vi "PopupList.vi"(8 "error in (no error)":errorcluster, 11 "BreadcrumbNavigation in":refnum<class "BreadcrumbNavigator.lvclass">) -> (0 "error out":errorcluster, 2 "SelectedItem":string, 3 "BreadcrumbNavigation out":refnum<class "BreadcrumbNavigator.lvclass">)   [LabVIEW 2015, in "BreadcrumbNavigator.lvclass"]
uses:
  BreadcrumbNavigator.lvclass
  <vilib>/Utility/miscctls.llb/LVPointTypeDef.ctl
  BreadcrumbNavigator.lvclass/BreadcrumbNavigator.ctl
  Read Strings[].vi
panel:
  in  "ItemList":i32(listbox)
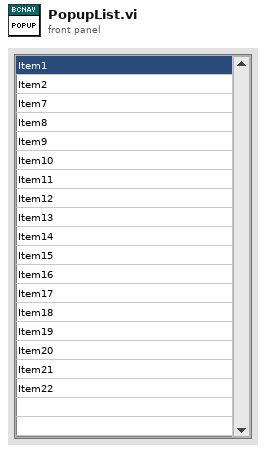
[diagram p1: front panel]
types:
  T1 = enum32{"Invalid", "Standard", "Closed", "Hidden", "Minimized", "Maximized"}
  T2 = typedef "LVPointTypeDef.ctl" = cluster{"Horizontal":i16, "Vertical":i16}
  T3 = typedef "LVRectTypeDef.ctl" = cluster{"Left":i16, "Top":i16, "Right":i16, "Bottom":i16}
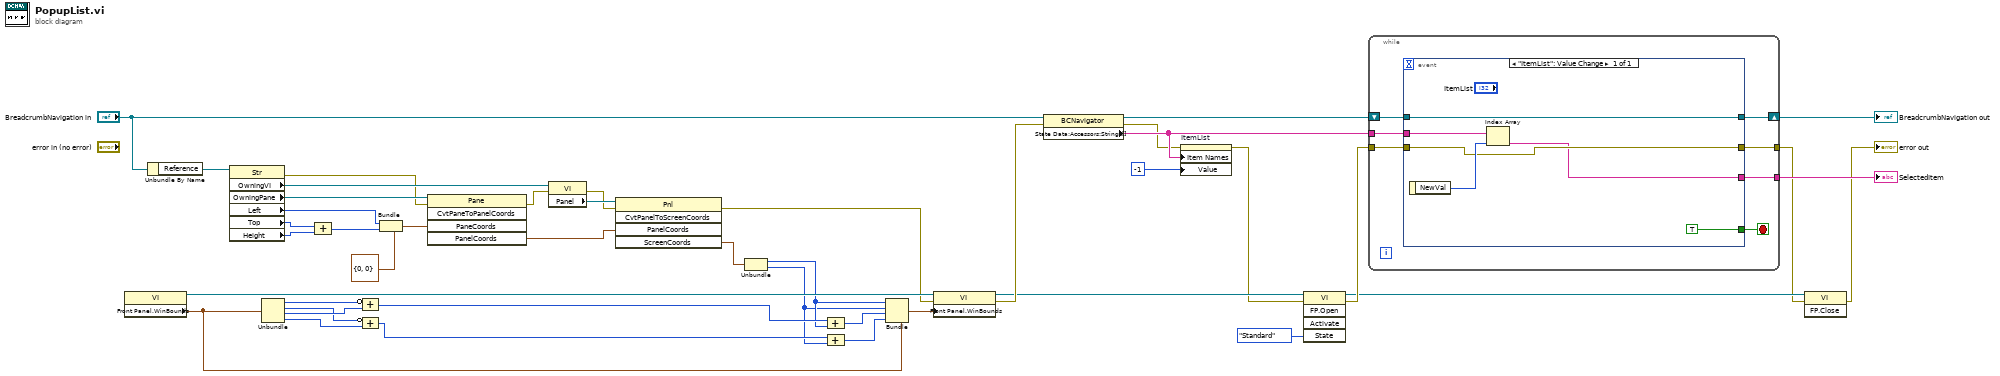
[diagram p0: block diagram]
diagram:
  n1 = property class="VI"() -> (reference out=w25:refnum<vi>, "Front Panel.WinBounds"=w27:T3)  [unwired: 2 in, 1 out]
  n2 = Unbundle By Name("BreadcrumbNavigation in") -> ("Reference"=w39:refnum<vi>)
  n3 = property class="Str"(reference=w39) -> (error out=w1:errorcluster, "OwningVI"=w31:refnum<vi>, "OwningPane"=w38:refnum<vi>, "Left"=w34:i32, "Top"=w37:i32, "Height"=w36:u32)  [unwired: 1 in, 1 out]
  n4 = Unbundle(w27) -> ("Left"=w13:i16, "Top"=w8:i16, "Right"=w12:i16, "Bottom"=w7:i16)
  n5 = Compound Arithmetic op=ADD(w37, w36) -> (w33:u32)
  n6 = Compound Arithmetic op=ADD(invert w13, w12) -> (w11:i16)
  n7 = Compound Arithmetic op=ADD(invert w8, w7) -> (w6:i16)
  n8 = Bundle(cluster=T2 {"Horizontal"=0, "Vertical"=0} ("Pane Coordinates"), "Horizontal"=w34, "Vertical"=w33) -> (w32:T2)
  n9 = invoke class="Pane" method="CvtPaneToPanelCoords"(reference=w38, error in=w1, "PaneCoords"=w32) -> (error out=w3:errorcluster, "PanelCoords"=w29:T2)  [unwired: 2 in, 3 out]
  n10 = property class="VI"(reference=w31, error in=w3) -> (error out=w2:errorcluster, "Panel"=w30:refnum<vi>)  [unwired: 1 out]
  n11 = invoke class="Pnl" method="CvtPanelToScreenCoords"(reference=w30, error in=w2, "PanelCoords"=w29) -> (error out=w20:errorcluster, "ScreenCoords"=w28:T2)  [unwired: 2 in, 3 out]
  n12 = Unbundle(w28) -> ("Horizontal"=w10:i16, "Vertical"=w5:i16)
  n13 = Compound Arithmetic op=ADD(w11, w10) -> (w9:i16)
  n14 = Compound Arithmetic op=ADD(w6, w5) -> (w4:i16)
  n15 = Bundle(cluster=w27, "Left"=w10, "Top"=w5, "Right"=w9, "Bottom"=w4) -> (w26:T3)
  n16 = property class="VI"(reference=w25, error in=w20, "Front Panel.WinBounds"=w26) -> (reference out=w23:refnum<vi>, error out=w24:errorcluster)
  n17 = property class="BCNavigator"(reference="BreadcrumbNavigation in", error in=w24) -> (reference out=w43:refnum<class "BreadcrumbNavigator.lvclass">, error out=w21:errorcluster, "State Data:Accessors:Strings[]"=w41:string[])
  n18 = property on="ItemList" class="LstBox (strict)"(error in=w21, "Item Names"=w41, "Value"=-1 ("ItemList")) -> (error out=w18:errorcluster)  [unwired: 1 in, 1 out]
  n19 = invoke class="VI" method="FP.Open"(reference=w23, error in=w18, "State"=T1."Standard") -> (reference out=w16:refnum<vi>, error out=w17:errorcluster)  [unwired: 2 in, 3 out]
  n20 = while {
    tunnel: [w46] -> w14
    tunnel: w17 -> [w50]
    shift-right: [w49] -> w44
    shift-left: w43 -> [w51]
    tunnel: w41 -> [w48]
    tunnel: [w45] -> w19
    stop <- w47 stop-if-true
    n21 = event shown="[0] \"ItemList\": Value Change" {
      selector: _ -> [_]
      dyn-events: _ -> [_]
      timeout: _ -> [_]
      tunnel: w51 -> [w57]
      tunnel: w50 -> [w53]
      tunnel: [w57] -> w49
      tunnel: w48 -> [w56]
      tunnel: [TRUE] -> w47
      tunnel: [w53] -> w46
      tunnel: [w52] -> w45
      event "ItemList": Value Change {
        n22 = event-data() -> ("NewVal"=w54:i32)  [unwired: 1 in]
        n23 = Index Array(array=w56, index=w54) -> (element=w52:string)
      }
    }
  }
  "BreadcrumbNavigation out" <- w44
  "SelectedItem" <- w19
  n24 = invoke class="VI" method="FP.Close"(reference=w16, error in=w14) -> (error out=→"error out":errorcluster)  [unwired: 1 in, 2 out]
